vi "Map_Update_Cell_Cost.vi"(6 "cell cost":dbl, 8 "error in (no error)":errorcluster, 9 "Y_map":i32, 10 "X_map":i32, 11 "Map_in":dbl[][](array[numeric])) -> (0 "error out":errorcluster, 3 "Map_out":dbl[][](array[numeric]))   [LabVIEW 2017]
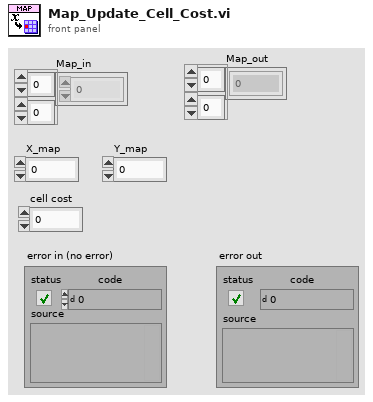
[diagram p1: front panel]
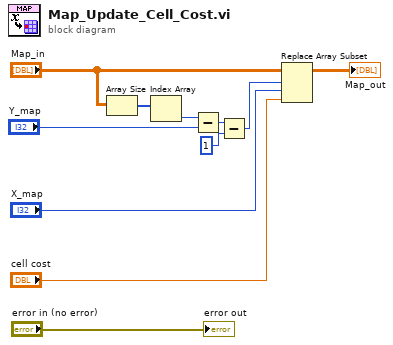
[diagram p0: block diagram]
diagram:
  n1 = Array Size(array="Map_in") -> (size(s)=w8:i32[])
  n2 = Index Array(array=w8) -> (element=w9:i32)  [unwired: 1 in]
  n3 = Subtract(x=w9, y="Y_map") -> (x-y=w5:i32)
  n4 = Subtract(x=w5, y=1) -> (x-y=w3:i32)
  n5 = Replace Array Subset(array="Map_in", new element="cell cost", index (row)=w3, index (col)="X_map") -> (→"Map_out":dbl[][])
  "error out" <- "error in (no error)"
